vi "LabView360-4.vi"() -> ()   [LabVIEW 2017]
panel:
  in  "停止 2":bool
  out "波形图":cluster{i32, i32, dbl[]}(graph)
  in  "停止":bool
  out "波形图表":T1(graph)
  # "通过帮助-查找范例来学习 Cluster 和接受各种\n数据类型的图标的使用"
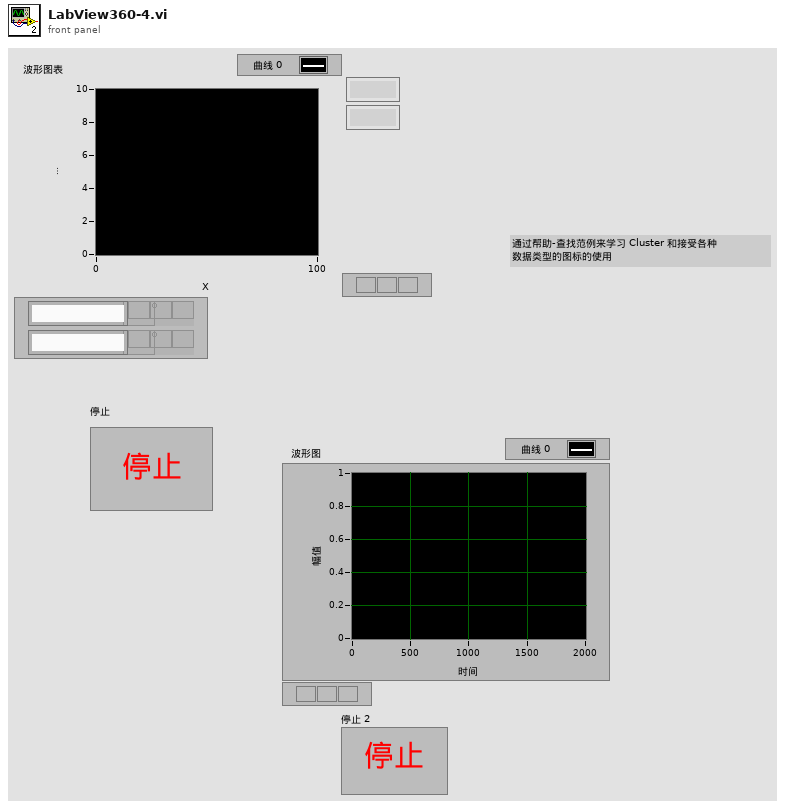
[diagram p1: front panel]
types:
  T1 = cluster{"number: 0 to 1":dbl, "number: 0 to 1":dbl}
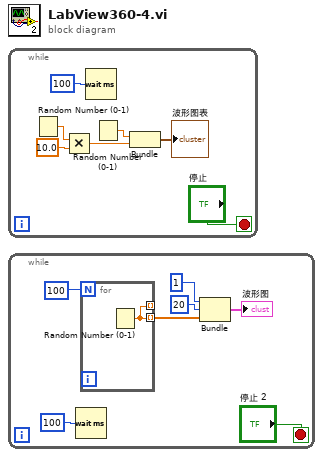
[diagram p0: block diagram]
diagram:
  n1 = while {
    stop <- "停止" stop-if-true
    n2 = Random Number (0-1)() -> (number: 0 to 1=w1:dbl)
    n3 = Multiply(x=w1, y=10.0) -> (x*y=w3:dbl)
    n4 = Wait (ms)(milliseconds to wait=u32 100 ("等待时间（毫秒）")) -> ()  [unwired: 1 out]
    n5 = Random Number (0-1)() -> (number: 0 to 1=w5:dbl)
    n6 = Bundle("number: 0 to 1"=w5, w3) -> (→"波形图表":cluster{"number: 0 to 1":dbl, dbl})  [unwired: 1 in]
  }
  n7 = while {
    stop <- "停止 2" stop-if-true
    n8 = Wait (ms)(milliseconds to wait=u32 100 ("等待时间（毫秒）")) -> ()  [unwired: 1 out]
    n9 = for {
      N: 100 -> [_]
      tunnel: [w15] -> _ mode=indexing
      tunnel: [w15] -> w12 mode=indexing
      n10 = Random Number (0-1)() -> (number: 0 to 1=w15:dbl)
    }
    n11 = Bundle(1, 20, w12) -> (→"波形图":cluster{i32, i32, dbl[]})  [unwired: 1 in]
  }
